vi "Update table.vi"() -> ()   [LabVIEW 2015]
uses:
  <vilib>/addons/database/Connection.llb/DB Tools Open Connec (Path).vi
  <vilib>/addons/database/Connection.llb/Conn Execute.vi
  <vilib>/addons/database/Recordset.llb/Rec Fetch Recordset Data (R).vi
  <vilib>/addons/database/Recordset.llb/Rec Destroy - Connection.vi
  <vilib>/addons/database/_DB Variant To Data/Database Variant To Data.xnode
  <vilib>/addons/database/NI_Database_API.lvlib
panel:
  in  "Name":string
  out "Array":string[][](array[string])
  in  "connection information":path
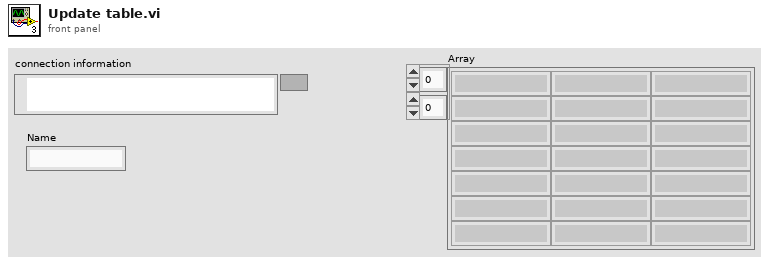
[diagram p1: front panel]
types:
  T1 = typedef "NI_Database_API.lvlib/Conn ObjectReference.ctl" = refnum<k1>
  T2 = typedef "NI_Database_API.lvlib/Rec ObjectReference.ctl" = refnum<k1>
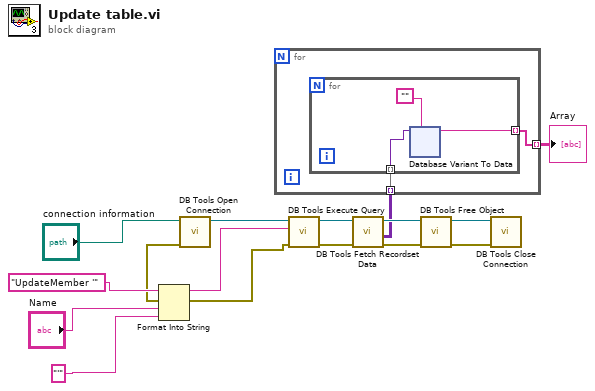
[diagram p0: block diagram]
diagram:
  n1 = call-poly <vilib>:"DB Tools Open Connection.vi"("connection information"="connection information") -> ("error out"=w3:errorcluster, "connection reference"=w13:T1)  [unwired: 7 in]
  n2 = Format Into String(initial string="UpdateMember '" ("SQL query"), error in=w3, "Name", "'") -> (resulting string=w6:string, error out=w4:errorcluster)  [unwired: 1 in]
  n3 = call-poly <vilib>:"DB Tools Execute Query.vi"("error in (no error)"=w4, "SQL query"=w6, "connection reference"=w13) -> ("error out"=w10:errorcluster, "recordset reference"=w12:T2)  [unwired: 5 in]
  n4 = call-poly <vilib>:"DB Tools Fetch Recordset Data.vi"("error in (no error)"=w10, "recordset reference"=w12) -> ("error out"=w9:errorcluster, "recordset data"=w8:variant[][], "recordset reference out"=w11:T2)  [unwired: 3 in]
  n5 = for {
    tunnel: [w18] -> w7 mode=indexing
    tunnel: w8 -> [w17] mode=indexing
    n6 = for {
      tunnel: [w21] -> w18 mode=indexing
      tunnel: w17 -> [w20] mode=indexing
      n7 = xnode "Database Variant To Data"("database variant"=w20, "type"="") -> ("data"=w21:string)  [unwired: 1 in, 1 out]
    }
  }
  "Array" <- w7
  n8 = call-poly <vilib>:"DB Tools Free Object.vi"("error in (no error)"=w9, "recordset reference"=w11) -> ("error out"=w16:errorcluster, "connection reference"=w15:T1)  [unwired: 8 in]
  n9 = call <vilib>:"DB Tools Close Connection.vi"("error in (no error)"=w16, "connection reference"=w15) -> ()  [unwired: 5 in, 1 out]
